vi "Startup.vi"   [LabVIEW 2016, in "Assert API Components.lvlib"]
uses:
  Assert API Components/Assert API Components.lvlib
  Assert Startup UI/Assert Startup UI/Assert Startup UI.lvclass
  C:/Program Files (x86)/National Instruments/LabVIEW 2016/vi.lib/ActorFramework/Actor/Actor.lvclass
  <vilib>/ActorFramework/Actor/Actor.lvclass
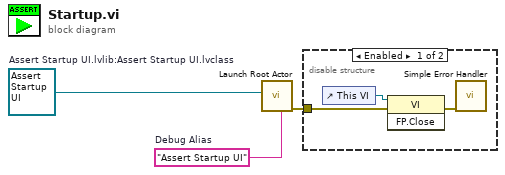
[diagram p0: block diagram]
diagram:
  w2 = "Assert Startup UI"  # Debug Alias
  w3 = refnum<class "Assert Startup UI.lvclass"> refnum  # Assert Startup UI.lvlib:Assert Startup UI.lvclass
  n1 = call <vilib>:"Launch Root Actor.vi"("Debug Alias"=w2, "Actor"=w3) -> ("error out"=w1:errorcluster)  [unwired: 8 in, 1 out]
  n2 = disable-structure shown="Enabled" {
    disable-tunnel: w1 -> [w5 _]
    frame Enabled {
      n3 = control-ref of="This VI"() -> (w6:refnum<vi>)
      n4 = invoke class="VI" method="FP.Close"(reference=w6, error in=w5) -> (error out=w4:errorcluster)  [unwired: 1 in, 2 out]
      n5 = call <vilib>:"Simple Error Handler.vi"("error in (no error)"=w4) -> ()  [unwired: 4 in, 5 out]
    }
    frame Disabled {
    }
  }
